vi "PSpeedControl.vi"(8 "Proportional Constant":dbl, 9 "Current Encoder Rates":dbl[](array[numeric]), 10 "Robot Max Rate":dbl, 11 "Targets":dbl[](array[numeric])) -> (0 "Motor Output 4":dbl, 1 "Motor Output 3":dbl, 2 "Motor Output 2":dbl, 3 "Motor Output 1":dbl)   [LabVIEW 2014]
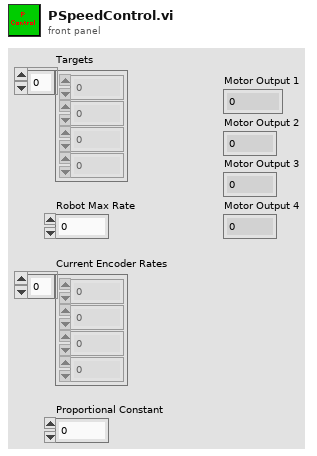
[diagram p1: front panel]
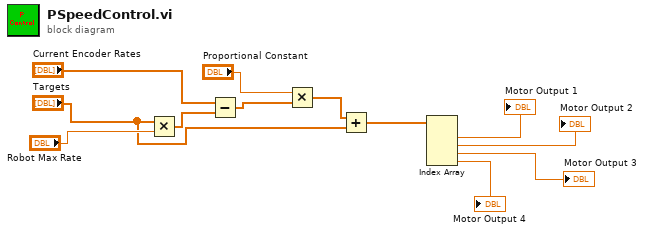
[diagram p0: block diagram]
diagram:
  n1 = Multiply(x="Targets", y="Robot Max Rate") -> (x*y=w10:dbl[])
  n2 = Subtract(x="Current Encoder Rates", y=w10) -> (x-y=w8:dbl[])
  n3 = Multiply(x="Proportional Constant", y=w8) -> (x*y=w6:dbl[])
  n4 = Add(x=w6, y="Targets") -> (x+y=w5:dbl[])
  n5 = Index Array(array=w5) -> (element #1=→"Motor Output 1":dbl, element #2=→"Motor Output 2":dbl, element #3=→"Motor Output 3":dbl, element #4=→"Motor Output 4":dbl)  [unwired: 4 in]
